vi "Read Register (U16).vi"(0 "session in":refnum<k21>, 5 "device":refnum<k21>="$DefaultDevices", 7 "register address":u32 format="%.0x", 11 "error in (no error)":errorcluster) -> (4 "session out":refnum<k21>, 6 "device out":refnum<k21>, 8 "next register address":u32 format="%.0x", 10 "data out":u16 format="%.0x", 15 "error out":errorcluster)   [LabVIEW 2020, in "SLSC.lvlib"]
doc: "Reads 16 bits from the given <B>register address</B> of the specified <B>device</B>."
uses:
  <vilib>/SLSC/SLSC.lvlib
  nislsclvapi.dll
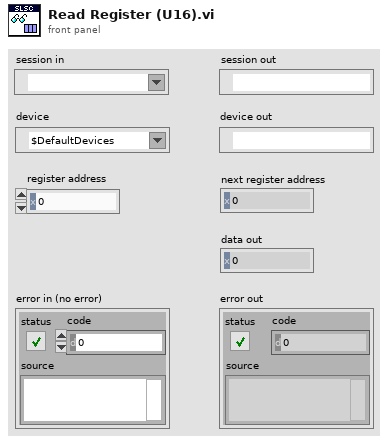
[diagram p1: front panel]
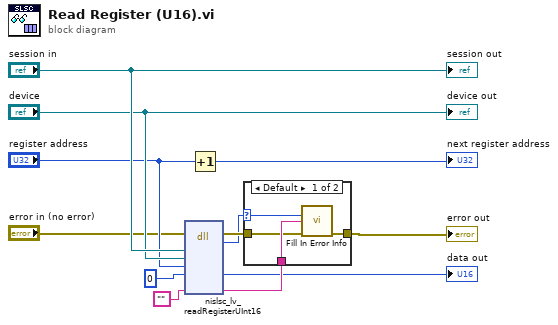
[diagram p0: block diagram]
diagram:
  n1 = dll-call lib="nislsclvapi.*" fn="nislsc_lv_readRegisterUInt16"(error in="error in (no error)", "session"="session in", "device"="device", "registerAddress"="register address", "data"=u16 0, "extendedErrorInfo"="") -> (error out=w10:errorcluster, "return type"=w9:i32, "data"=→"data out":u16, "extendedErrorInfo"=w11:string)  [unwired: 7 in, 1 out]
  n2 = Increment(x="register address") -> (x+1=→"next register address":u32)
  n3 = case shown="Default" w9 {
    selector: w9 -> [w16 _]
    tunnel: w11 -> [w15 _]
    tunnel: w10 -> [w14 w17]
    tunnel: [w13 w17] -> w2
    frame Default {
      n4 = call <vilib>:"Fill In Error Info.vi"("status code"=w16, "extended error info"=w15, "error in"=w14) -> ("error out"=w13:errorcluster)  [unwired: 12 in]
    }
    frame 0 {
    }
  }
  "error out" <- w2
  "session out" <- "session in"
  "device out" <- "device"
